vi "StopReading2.vi"() -> ()   [LabVIEW 2020]
panel:
  out "Stop":bool
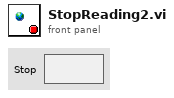
[diagram p1: front panel]
diagram:
